vi "run_database.vi"() -> ()   [LabVIEW 2011]
uses:
  <vilib>/addons/database/Connection.llb/DB Tools Open Connec (String).vi
  Dependencies/global.vi
  <vilib>/addons/database/NI_Database_API.lvlib
panel:
  out "Connection Error 4":errorcluster
  out "# Received Data from weather_station.vi":u64
  out "LabVIEW Started at":string
  out "Database Backup Path (remote PC)":path
  out "Backup Error Msg (remote PC)":string
  out "In Progress":bool
  out "Connection Error 3":errorcluster
  out "# Received Data from counter.vi":u64
  out "Dequeue Rate (per second)":dbl
  out "# Elements in Real-time Queue":u64
  out "# Received Data from plc.vi":u64
  out "Connection Error 2":errorcluster
  out "# of Dequeues (total)":u64
  in  "Pause Database Writing (s)":dbl=5.0
  in  "Backup Interval (hour)":dbl=24.0
  out "Backup Error Msg (local PC)":string
  out "Database Backup Path (local PC)":path
  out "Dequeue Paused":bool
  out "# of Backups":u64
  out "Next Backup Dues in (s):":u64 caption="Elapsed Time (s)"
  out "Database Path":path
  out "# Elements in Database Queue":u64
  out "Dequeue Error":errorcluster
  out "Database Access Error":errorcluster
  out "# Received Data from mote.vi":u64
  out "Connection Error":errorcluster
  # "Receive data from motes and Enqueue"
  # "Dequeue and write to database"
  # "Backup database"
  # "Receive data from plcs and Enqueue"
  # "Receive data from people counter and Enqueue"
  # "Receive data from weather station"
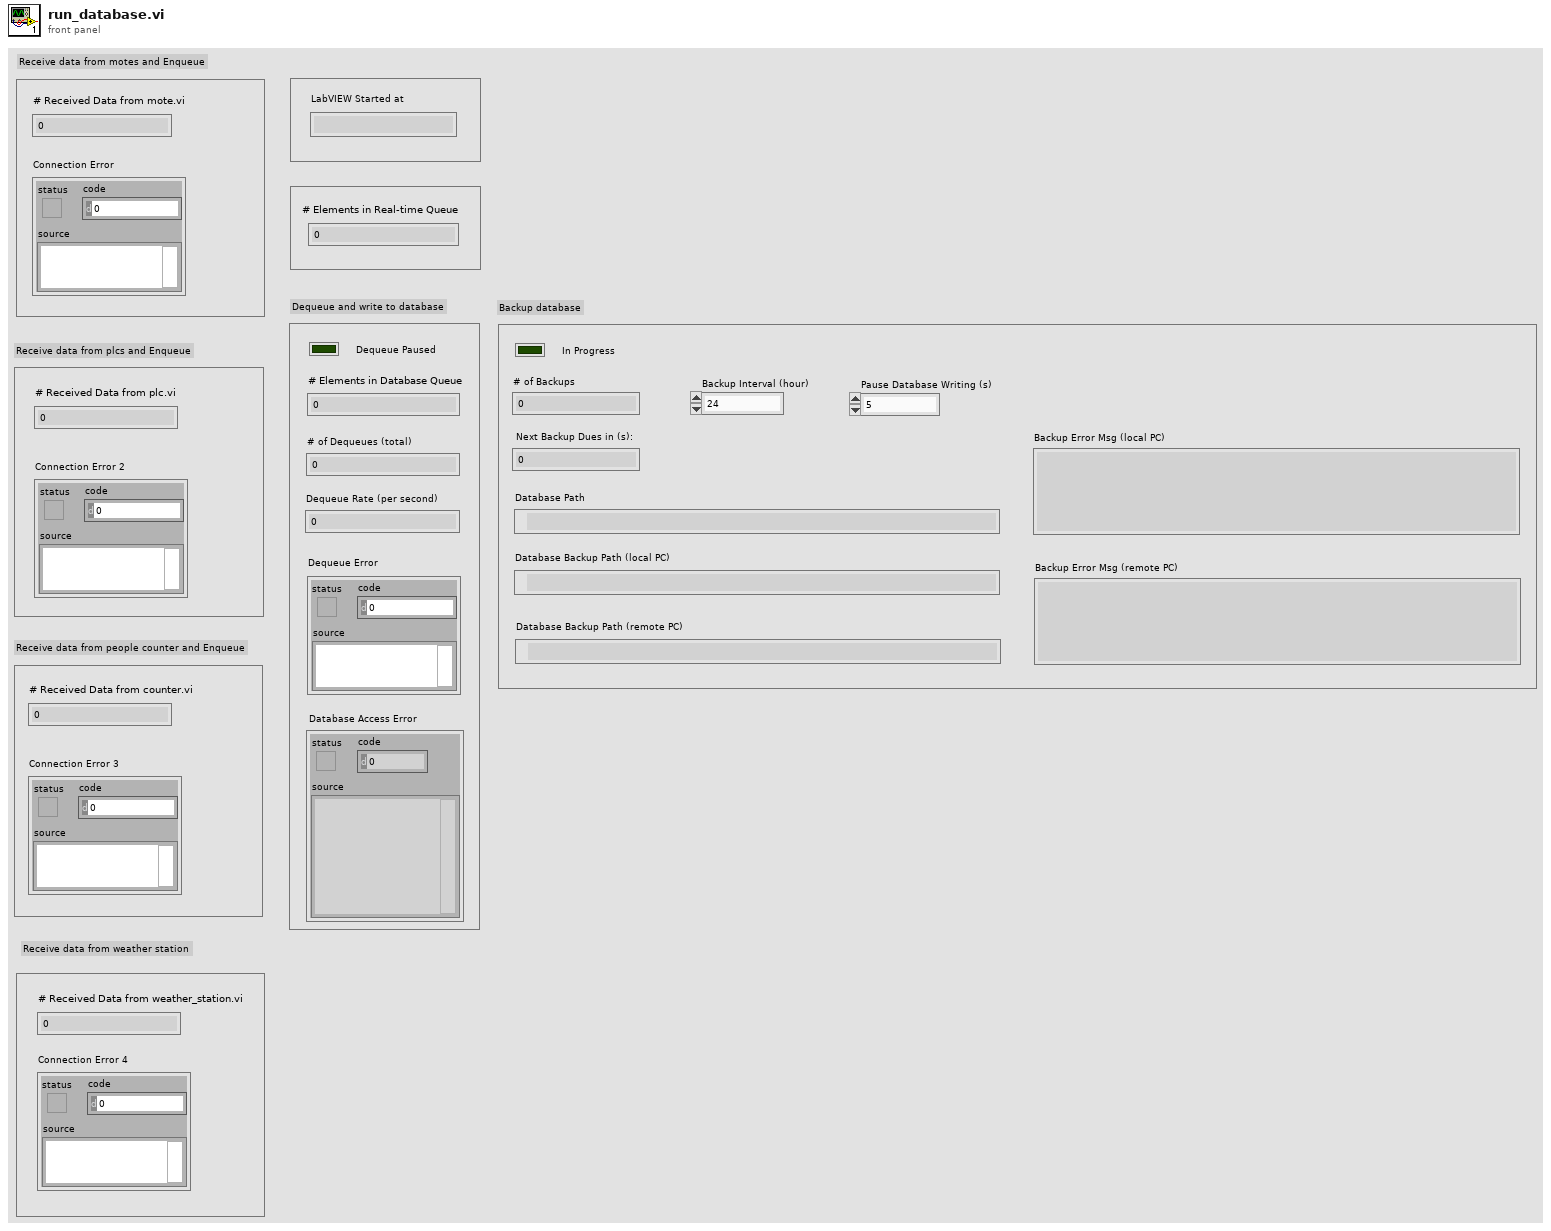
[diagram p1: front panel]
types:
  T1 = enum16{"Read", "Write", "ReadWrite", "BufferedRead", "BufferedReadWrite"}
  T2 = cluster{string, string, string, string, string, string, string, string}
  T3 = cluster{string, "output string":string, "output string":string, "output string":string, "output string":string, "output string":string, "output string":string, "output string":string}
  T4 = typedef "NI_Database_API.lvlib/Conn ObjectReference.ctl" = refnum<k1>
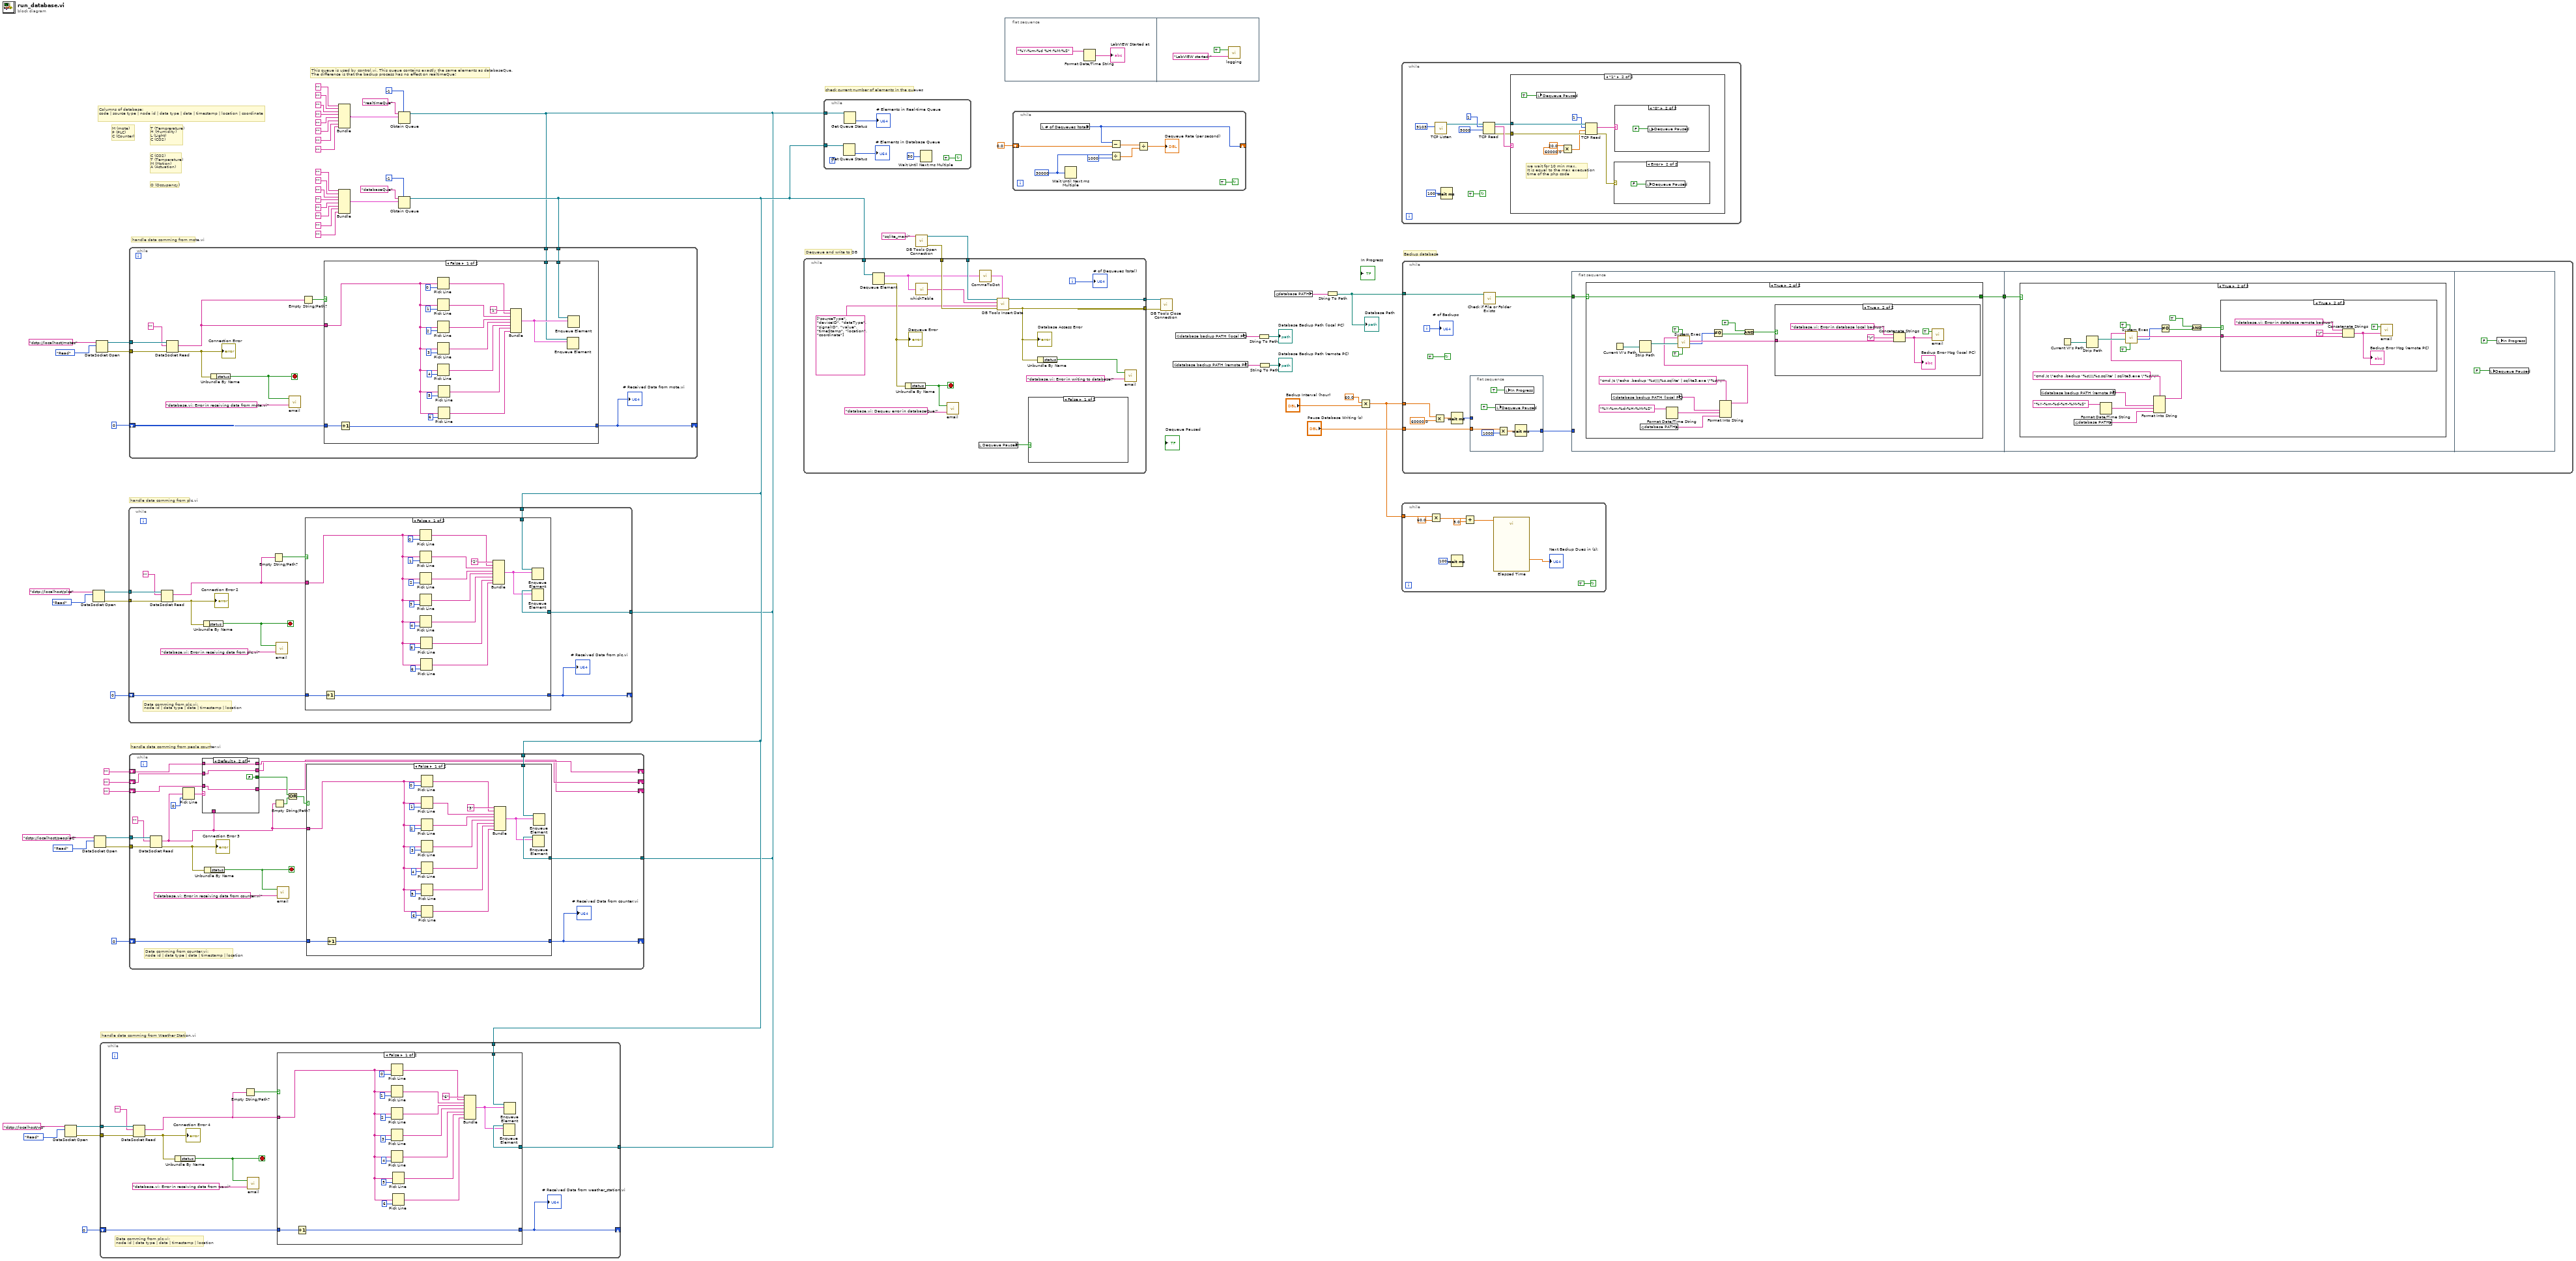
[diagram p0: block diagram]
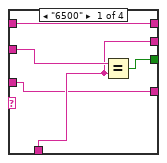
[diagram p6: hidden frame]
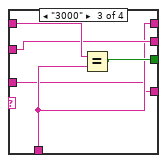
[diagram p7: hidden frame]
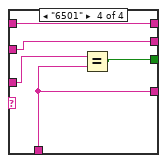
[diagram p8: hidden frame]
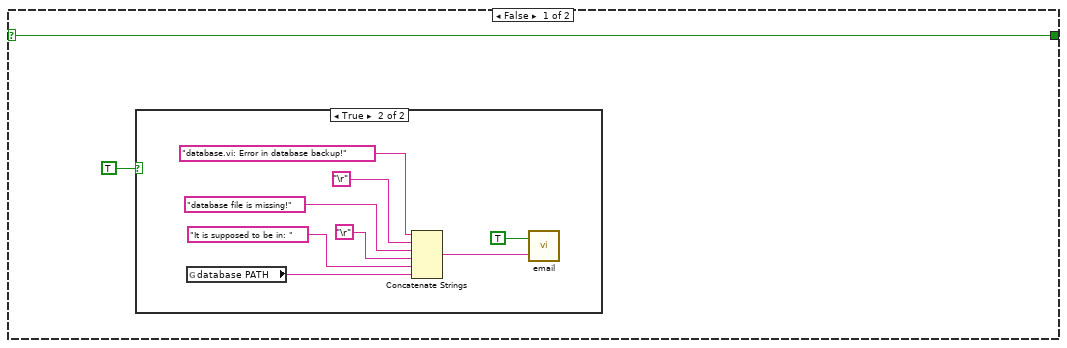
[diagram p11: hidden frame]
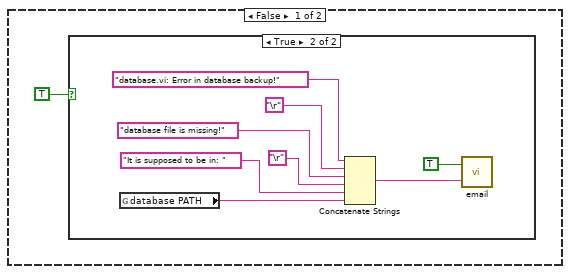
[diagram p14: hidden frame]
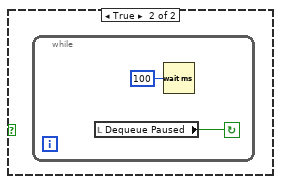
[diagram p17: hidden frame]
diagram:
  # "handle data comming from Weather Station.vi"
  # "handle data comming from peole counter.vi"
  # "O (Occupancy)"
  # "C (CO2)\nT (Temperature)\nM (Motion)\nA (Actuation)"
  # "This queue is used by control.vi. This queue contains exactly the same elements as databaseQue.\nThe difference is that the backup process has no effect on realtimeQue!"
  # "handle data comming from plc.vi"
  # "handle data comming from mote.vi"
  # "Backup database"
  # "Dequeue and write to DB"
  # "check current number of elements in the queues"
  # "M (mote)\nP (PLC)\nC (Counter)"
  # "T (Temprerature)\nH (Humidity)\nL (Light)\nC (CO2)"
  # "Columns of database:\ncode | source type | node id | data type | data | timestamp | location | coordinate"
  n1 = DataSocket Open(10:T1."Read" ("mode"), 11:"dstp://localhost/ws" ("URL 3")) -> (0:w5:errorcluster, 3:w4:refnum<k13>)  [unwired: 2 in]
  n2 = DataSocket Open(10:T1."Read" ("mode"), 11:"dstp://localhost/plcs" ("URL 3")) -> (0:w46:errorcluster, 3:w45:refnum<k13>)  [unwired: 2 in]
  n3 = DataSocket Open(10:T1."Read" ("mode"), 11:"dstp://localhost/peopleC" ("URL 3")) -> (0:w37:errorcluster, 3:w38:refnum<k13>)  [unwired: 2 in]
  n4 = DataSocket Open(10:T1."Read" ("mode"), 11:"dstp://localhost/motes" ("URL 3")) -> (0:w50:errorcluster, 3:w49:refnum<k13>)  [unwired: 2 in]
  n5 = Bundle("", "", "", "", "", "", "", "") -> (w14:T2)  [unwired: 1 in]
  n6 = Bundle("", "", "", "", "", "", "", "") -> (w13:T2)  [unwired: 1 in]
  n7 = Obtain Queue(max queue size (-1, unlimited)=-1, name (unnamed)="realtimeQue", element data type=w14) -> (queue out=w1:refnum<queue>)  [unwired: 2 in, 2 out]
  n8 = Obtain Queue(max queue size (-1, unlimited)=-1, name (unnamed)="databaseQue", element data type=w13) -> (queue out=w2:refnum<queue>)  [unwired: 2 in, 2 out]
  n9 = while {
    tunnel: w5 -> [w75]
    tunnel: w4 -> [w74]
    tunnel: w2 -> [w72]
    tunnel: w1 -> [w70]
    shift-right: [w65] -> _
    shift-left: u64 0 -> [w66]
    stop <- w67 stop-if-true
    # "Data comming from plc.vi:\nnode id | data type | data | timestamp | location"
    n10 = DataSocket Read(8:w75, 10:"", 11:w74) -> (0:w73:errorcluster, 2:w68:string)  [unwired: 2 in, 5 out]
    "Connection Error 4" <- w73
    n11 = Unbundle By Name(w73) -> ("status"=w67:bool)
    n12 = Empty String/Path?(string/path=w68) -> (empty?=w69:bool)
    n13 = call "email.vi"("Body"="database.vi: Error in receiving data from ws.vi", "Enable"=w67) -> ()  [unwired: 1 in]
    n14 = case shown="False" w69 {
      tunnel: w72 -> [w96 _]
      tunnel: w68 -> [w80 _]
      tunnel: w70 -> [w90 _]
      tunnel: w66 -> [w88 w97]
      tunnel: [w87 w97] -> w65
      frame False {
        n15 = Increment(x=w88) -> (x+1=w87:u64)
        n16 = Pick Line(multi-line string=w80, line index=0) -> (output string=w76:string)  [unwired: 1 in]
        n17 = Pick Line(multi-line string=w80, line index=1) -> (output string=w86:string)  [unwired: 1 in]
        n18 = Pick Line(multi-line string=w80, line index=2) -> (output string=w85:string)  [unwired: 1 in]
        n19 = Pick Line(multi-line string=w80, line index=3) -> (output string=w84:string)  [unwired: 1 in]
        n20 = Pick Line(multi-line string=w80, line index=4) -> (output string=w83:string)  [unwired: 1 in]
        n21 = Pick Line(multi-line string=w80, line index=5) -> (output string=w79:string)  [unwired: 1 in]
        n22 = Pick Line(multi-line string=w80, line index=6) -> (output string=w78:string)  [unwired: 1 in]
        n23 = Bundle("6", "output string"=w76, "output string"=w86, "output string"=w85, "output string"=w84, "output string"=w83, "output string"=w79, "output string"=w78) -> (w89:T3)  [unwired: 1 in]
        n24 = Enqueue Element(queue=w90, element=w89) -> ()  [unwired: 2 in, 3 out]
        n25 = Enqueue Element(queue=w96, element=w89) -> ()  [unwired: 2 in, 3 out]
      }
      frame True {
      }
    }
    "# Received Data from weather_station.vi" <- w65
  }
  n26 = while {
    tunnel: w46 -> [w109]
    tunnel: w45 -> [w108]
    tunnel: w2 -> [w106]
    tunnel: w1 -> [w104]
    shift-right: [w99] -> _
    shift-left: u64 0 -> [w100]
    stop <- w101 stop-if-true
    # "Data comming from plc.vi:\nnode id | data type | data | timestamp | location"
    n27 = DataSocket Read(8:w109, 10:"", 11:w108) -> (0:w107:errorcluster, 2:w102:string)  [unwired: 2 in, 5 out]
    "Connection Error 2" <- w107
    n28 = Unbundle By Name(w107) -> ("status"=w101:bool)
    n29 = Empty String/Path?(string/path=w102) -> (empty?=w103:bool)
    n30 = call "email.vi"("Body"="database.vi: Error in receiving data from plc.vi", "Enable"=w101) -> ()  [unwired: 1 in]
    n31 = case shown="False" w103 {
      tunnel: w106 -> [w130 _]
      tunnel: w102 -> [w114 _]
      tunnel: w104 -> [w124 _]
      tunnel: w100 -> [w122 w131]
      tunnel: [w121 w131] -> w99
      frame False {
        n32 = Increment(x=w122) -> (x+1=w121:u64)
        n33 = Pick Line(multi-line string=w114, line index=0) -> (output string=w110:string)  [unwired: 1 in]
        n34 = Pick Line(multi-line string=w114, line index=1) -> (output string=w120:string)  [unwired: 1 in]
        n35 = Pick Line(multi-line string=w114, line index=2) -> (output string=w119:string)  [unwired: 1 in]
        n36 = Pick Line(multi-line string=w114, line index=3) -> (output string=w118:string)  [unwired: 1 in]
        n37 = Pick Line(multi-line string=w114, line index=4) -> (output string=w117:string)  [unwired: 1 in]
        n38 = Pick Line(multi-line string=w114, line index=5) -> (output string=w113:string)  [unwired: 1 in]
        n39 = Pick Line(multi-line string=w114, line index=6) -> (output string=w112:string)  [unwired: 1 in]
        n40 = Bundle("2", "output string"=w110, "output string"=w120, "output string"=w119, "output string"=w118, "output string"=w117, "output string"=w113, "output string"=w112) -> (w123:T3)  [unwired: 1 in]
        n41 = Enqueue Element(queue=w124, element=w123) -> ()  [unwired: 2 in, 3 out]
        n42 = Enqueue Element(queue=w130, element=w123) -> ()  [unwired: 2 in, 3 out]
      }
      frame True {
      }
    }
    "# Received Data from plc.vi" <- w99
  }
  n43 = while {
    tunnel: w50 -> [w143]
    tunnel: w49 -> [w142]
    tunnel: w2 -> [w140]
    tunnel: w1 -> [w139]
    shift-right: [w136] -> _
    shift-left: u64 0 -> [w137]
    stop <- w138 stop-if-true
    n44 = DataSocket Read(8:w143, 10:"", 11:w142) -> (0:w141:errorcluster, 2:w132:string)  [unwired: 2 in, 5 out]
    "Connection Error" <- w141
    n45 = Unbundle By Name(w141) -> ("status"=w138:bool)
    n46 = call "email.vi"("Body"="database.vi: Error in receiving data from mote.vi", "Enable"=w138) -> ()  [unwired: 1 in]
    n47 = Empty String/Path?(string/path=w132) -> (empty?=w134:bool)
    n48 = case shown="False" w134 {
      tunnel: w140 -> [w148 _]
      tunnel: w132 -> [w146 _]
      tunnel: w139 -> [w147 _]
      tunnel: [w164 w165] -> w136
      tunnel: w137 -> [w163 w165]
      frame False {
        n49 = Increment(x=w163) -> (x+1=w164:u64)
        n50 = Pick Line(multi-line string=w146, line index=0) -> (output string=w144:string)  [unwired: 1 in]
        n51 = Pick Line(multi-line string=w146, line index=1) -> (output string=w156:string)  [unwired: 1 in]
        n52 = Pick Line(multi-line string=w146, line index=2) -> (output string=w155:string)  [unwired: 1 in]
        n53 = Pick Line(multi-line string=w146, line index=3) -> (output string=w154:string)  [unwired: 1 in]
        n54 = Pick Line(multi-line string=w146, line index=4) -> (output string=w153:string)  [unwired: 1 in]
        n55 = Pick Line(multi-line string=w146, line index=5) -> (output string=w150:string)  [unwired: 1 in]
        n56 = Pick Line(multi-line string=w146, line index=6) -> (output string=w149:string)  [unwired: 1 in]
        n57 = Bundle("1", "output string"=w144, "output string"=w156, "output string"=w155, "output string"=w154, "output string"=w153, "output string"=w150, "output string"=w149) -> (w157:T3)  [unwired: 1 in]
        n58 = Enqueue Element(queue=w147, element=w157) -> ()  [unwired: 2 in, 3 out]
        n59 = Enqueue Element(queue=w148, element=w157) -> ()  [unwired: 2 in, 3 out]
      }
      frame True {
      }
    }
    "# Received Data from mote.vi" <- w136
  }
  n60 = while {
    tunnel: w37 -> [w187]
    tunnel: w38 -> [w186]
    tunnel: w2 -> [w184]
    tunnel: w1 -> [w182]
    shift-right: [w179] -> _
    shift-left: u64 0 -> [w180]
    shift-right: [w169] -> _
    shift-left: "" -> [w173]
    shift-right: [w168] -> _
    shift-left: "" -> [w170]
    shift-right: [w166] -> _
    shift-left: "" -> [w167]
    stop <- w181 stop-if-true
    # "Data comming from counter.vi:\nnode id | data type | data | timestamp | location"
    n61 = DataSocket Read(8:w187, 10:"", 11:w186) -> (0:w185:errorcluster, 2:w172:string)  [unwired: 2 in, 5 out]
    "Connection Error 3" <- w185
    n62 = Pick Line(multi-line string=w172, line index=0) -> (output string=w174:string)  [unwired: 1 in]
    n63 = case shown="Default" w174 {
      tunnel: w173 -> [w191 w196 w200 w204]
      tunnel: w172 -> [w189 _ w198 w202]
      tunnel: [w192 FALSE w201 w206] -> w171
      tunnel: w170 -> [w190 w195 w199 w205]
      tunnel: [w191 w196 w198 w204] -> w169
      tunnel: [w189 w195 w199 w205] -> w168
      tunnel: w167 -> [w188 w193 w197 w203]
      tunnel: [w188 w193 w197 w202] -> w166
      frame "6500" {
        n64 = Equal?(x=w190, y=w189) -> (x = y?=w192:bool)
      }
      frame Default {
      }
      frame "3000" {
        n65 = Equal?(x=w200, y=w198) -> (x = y?=w201:bool)
      }
      frame "6501" {
        n66 = Equal?(x=w203, y=w202) -> (x = y?=w206:bool)
      }
    }
    n67 = Unbundle By Name(w185) -> ("status"=w181:bool)
    n68 = Empty String/Path?(string/path=w172) -> (empty?=w177:bool)
    n69 = call "email.vi"("Body"="database.vi: Error in receiving data from counter.vi", "Enable"=w181) -> ()  [unwired: 1 in]
    n70 = Or(x=w171, y=w177) -> (x .or. y?=w176:bool)
    n71 = case shown="False" w176 {
      tunnel: w184 -> [w227 _]
      tunnel: w172 -> [w211 _]
      tunnel: w182 -> [w221 _]
      tunnel: w180 -> [w219 w228]
      tunnel: [w218 w228] -> w179
      frame False {
        n72 = Increment(x=w219) -> (x+1=w218:u64)
        n73 = Pick Line(multi-line string=w211, line index=0) -> (output string=w207:string)  [unwired: 1 in]
        n74 = Pick Line(multi-line string=w211, line index=1) -> (output string=w217:string)  [unwired: 1 in]
        n75 = Pick Line(multi-line string=w211, line index=2) -> (output string=w216:string)  [unwired: 1 in]
        n76 = Pick Line(multi-line string=w211, line index=3) -> (output string=w215:string)  [unwired: 1 in]
        n77 = Pick Line(multi-line string=w211, line index=4) -> (output string=w214:string)  [unwired: 1 in]
        n78 = Pick Line(multi-line string=w211, line index=5) -> (output string=w210:string)  [unwired: 1 in]
        n79 = Pick Line(multi-line string=w211, line index=6) -> (output string=w209:string)  [unwired: 1 in]
        n80 = Bundle("3", "output string"=w207, "output string"=w217, "output string"=w216, "output string"=w215, "output string"=w214, "output string"=w210, "output string"=w209) -> (w220:T3)  [unwired: 1 in]
        n81 = Enqueue Element(queue=w221, element=w220) -> ()  [unwired: 2 in, 3 out]
        n82 = Enqueue Element(queue=w227, element=w220) -> ()  [unwired: 2 in, 3 out]
      }
      frame True {
      }
    }
    "# Received Data from counter.vi" <- w179
  }
  n83 = while {
    tunnel: w2 -> [w234]
    tunnel: w1 -> [w230]
    stop <- TRUE continue-if-true
    n84 = Get Queue Status(queue=w234) -> (# elements in queue=→"# Elements in Database Queue":i32)  [unwired: 2 in, 7 out]
    n85 = Get Queue Status(queue=w230) -> (# elements in queue=→"# Elements in Real-time Queue":i32)  [unwired: 2 in, 7 out]
    n86 = Wait Until Next ms Multiple(millisecond multiple=u32 50) -> ()  [unwired: 1 out]
  }
  n87 = call-poly <vilib>:"DB Tools Open Connection.vi"("connection information"="sqlite_mani") -> ("error out"=w56:errorcluster, "connection reference"=w59:T4)  [unwired: 7 in]
  n88 = while {
    tunnel: w59 -> [w249]
    tunnel: [w250] -> w58
    tunnel: [w240] -> w57
    tunnel: w56 -> [w248]
    tunnel: w2 -> [w247]
    i -> [w243]
    stop <- w241 stop-if-true
    n89 = Dequeue Element(queue=w247) -> (element=w236:T2, error out=w246:errorcluster)  [unwired: 2 in, 2 out]
    "Dequeue Error" <- w246
    n90 = Unbundle By Name(w246) -> ("status"=w241:bool)
    n91 = call "whichTable.vi"("output cluster"=w236) -> ("String"=w242:string)
    n92 = call "email.vi"("Body"="database.vi: Dequeu error in databaseQue!", "Enable"=w241) -> ()  [unwired: 1 in]
    n93 = local read "Dequeue Paused"() -> (w244:bool)
    n94 = call "CommaToDot.vi"("Input"=w236) -> ("Output"=w235:T2)
    n95 = call <vilib>:"DB Tools Insert Data.vi"("data"=w235, "error in (no error)"=w248, "columns"=string[] ["sourceType", "deviceID", "dataType", "signalID", "value", "timeStamp", "location", "coordinate"], "table"=w242, "connection reference"=w249) -> ("error out"=w240:errorcluster, "connection reference out"=w250:T4)  [unwired: 5 in]
    "Database Access Error" <- w240
    n96 = case shown="False" w244 {
      frame False {
      }
      frame True {
        n97 = while {
          stop <- w251 continue-if-true
          n98 = local read "Dequeue Paused"() -> (w251:bool)
          n99 = Wait (ms)(milliseconds to wait=u32 100) -> ()  [unwired: 1 out]
        }
      }
    }
    n100 = Unbundle By Name(w240) -> ("status"=w239:bool)
    n101 = call "email.vi"("Body"="database.vi: Error in writing to database!", "Enable"=w239) -> ()  [unwired: 1 in]
    "# of Dequeues (total)" <- w243
  }
  n102 = flat-sequence {
    frame #0 {
      n103 = Format Date/Time String(time format string (%c)="%Y-%m-%d %H:%M:%S") -> (date/time string=→"LabVIEW Started at":string)  [unwired: 2 in]
    }
    frame #1 {
      n104 = call "logging.vi"("data"="LabVIEW started.", "Boolean"=TRUE) -> ()  [unwired: 1 in]
    }
  }
  n105 = while {
    shift-right: [w262] -> _
    shift-left: 0.0 -> [w263]
    stop <- TRUE continue-if-true
    w259 = u32 30000 ("millisecond multiple")
    n106 = local read "# of Dequeues (total)"() -> (w262:u64)
    n107 = Wait Until Next ms Multiple(millisecond multiple=w259) -> ()  [unwired: 1 out]
    n108 = Subtract(x=w262, y=w263) -> (x-y=w261:dbl)
    n109 = Divide(x=w259, y=u32 1000) -> (x/y=w257:dbl)
    n110 = Divide(x=w261, y=w257) -> (x/y=→"Dequeue Rate (per second)":dbl)
  }
  n111 = call <vilib>:"DB Tools Close Connection.vi"("error in (no error)"=w57, "connection reference"=w58) -> ()  [unwired: 5 in, 1 out]
  n112 = global read "global.vi" "database backup PATH (remote PC)"() -> (w11:string)
  n113 = global read "global.vi" "database backup PATH (local PC)"() -> (w53:string)
  n114 = String To Path(string=w53) -> (path=→"Database Backup Path (local PC)":path)
  n115 = String To Path(string=w11) -> (path=→"Database Backup Path (remote PC)":path)
  n116 = global read "global.vi" "database PATH"() -> (w55:string)
  n117 = String To Path(string=w55) -> (path=w54:path)
  "Database Path" <- w54
  n118 = Multiply(x=60.0, y="Backup Interval (hour)") -> (x*y=w31:dbl)
  n119 = while {
    stop <- TRUE continue-if-true
    n120 = call <vilib>:"TCP Listen.vi"("port"=u16 9103) -> ("connection ID"=w268:refnum<k5>)  [unwired: 6 in, 4 out]
    n121 = Wait (ms)(milliseconds to wait=u32 100) -> ()  [unwired: 1 out]
    n122 = TCP Read(connection ID=w268, bytes to read=1, 9:5000 ("timeout ms (25000)")) -> (connection ID out=w266:refnum<k5>, data out=w267:string, error out=w265:errorcluster)  [unwired: 2 in]
    n123 = case shown="\"1\"" w267 {
      tunnel: w266 -> [_ w282]
      tunnel: w265 -> [_ w281]
      frame "0", Default {
      }
      frame "1" {
        # "we wait for 10 min max.\nIt is equal to the max execuation\ntime of the php code"
        n124 = local write "Dequeue Paused"(TRUE ("Backup in Progress")) -> ()
        n125 = Multiply(x=20.0, y=60000.0) -> (x*y=w274:dbl)
        n126 = TCP Read(connection ID=w282, bytes to read=1, error in (no error)=w281, 9:w274) -> (data out=w278:string, error out=w277:errorcluster)  [unwired: 1 in, 1 out]
        n127 = case shown="Error" w277 {
          frame No Error {
          }
          frame Error {
            n128 = local write "Dequeue Paused"(FALSE ("Backup in Progress")) -> ()
          }
        }
        n129 = case shown="\"0\"" w278 {
          frame "1", Default {
          }
          frame "0" {
            n130 = local write "Dequeue Paused"(FALSE ("Backup in Progress")) -> ()
          }
        }
      }
    }
  }
  n131 = while {
    tunnel: w31 -> [w290]
    stop <- TRUE continue-if-true
    n132 = Multiply(x=w290, y=60.0) -> (x*y=w287:dbl)
    n133 = Wait (ms)(milliseconds to wait=u32 100) -> ()  [unwired: 1 out]
    n134 = Add(x=w287, y=5.0) -> (x+y=w288:dbl)
    n135 = call "Elapsed Time"("Time Target (s)"=w288) -> ("Elapsed Time (s)"=→"Next Backup Dues in (s):":dbl)  [unwired: 11 in, 7 out]
  }
  n136 = while {
    tunnel: w54 -> [w302]
    tunnel: w31 -> [w296]
    tunnel: "Pause Database Writing (s)" -> [w295]
    i -> [w294]
    stop <- TRUE continue-if-true
    n137 = Multiply(x=w296, y=60000.0) -> (x*y=w297:dbl)
    n138 = Wait (ms)(milliseconds to wait=w297) -> (millisecond timer value=w301:u32)
    n139 = flat-sequence {
      tunnel: w301 -> [_]
      tunnel: [w309] -> w300
      tunnel: w295 -> [w307]
      frame #0 {
        n140 = local write "Dequeue Paused"(TRUE ("Pause Write to DB")) -> ()
        n141 = Multiply(x=w307, y=u32 1000) -> (x*y=w308:dbl)
        n142 = local write "In Progress"(TRUE ("In Progress")) -> ()
        n143 = Wait (ms)(milliseconds to wait=w308) -> (millisecond timer value=w309:u32)
      }
    }
    n144 = call <vilib>:"Check if File or Folder Exists.vi"("path"=w302) -> ("file or folder exists?"=w298:bool)  [unwired: 8 in, 2 out]
    n145 = flat-sequence {
      tunnel: w300 -> [_]
      tunnel: w298 -> [w311]
      tunnel: [w310] -> w293
      tunnel: w293 -> [w343]
      frame #0 {
        n146 = case shown="True" w311 {
          selector: w311 -> [w312 w322]
          tunnel: [w312 w322] -> w310
          frame False {
            n147 = case shown="True" TRUE {
              frame False {
              }
              frame True {
                n148 = global read "global.vi" "database PATH"() -> (w316:string)
                n149 = Concatenate Strings("database.vi: Error in database backup!", "\r", "database file is missing!", "\r", "It is supposed to be in: ", w316) -> (w314:string)
                n150 = call "email.vi"("Body"=w314, "Enable"=TRUE) -> ()  [unwired: 1 in]
              }
            }
          }
          frame True {
            n151 = global read "global.vi" "database backup PATH (local PC)"() -> (w326:string)
            n152 = Current VI's Path() -> (path=w333:path)
            n153 = Strip Path(path=w333) -> (stripped path=w332:path)  [unwired: 1 out]
            n154 = global read "global.vi" "database PATH"() -> (w328:string)
            n155 = Format Date/Time String(time format string (%c)="%Y-%m-%d-%H-%M-%S") -> (date/time string=w327:string)  [unwired: 2 in]
            n156 = Format Into String(format string="cmd /c \"echo .backup '%s\\\\%s.sqlite' | sqlite3.exe \"%s\"\"", w326, w327, w328) -> (resulting string=w323:string)  [unwired: 2 in, 1 out]
            n157 = call <vilib>:"System Exec.vi"("run minimized? (F)"=TRUE, "wait until completion? (T)"=TRUE, "working directory"=w332, "command line"=w323) -> ("return code"=w330:i32, "standard error"=w331:string)  [unwired: 4 in, 2 out]
            n158 = Not Equal To 0?(x=w330) -> (x != 0?=w329:bool)
            n159 = And(x=TRUE, y=w329) -> (x .and. y?=w337:bool)
            n160 = case shown="True" w337 {
              tunnel: w331 -> [_ w340]
              frame False {
              }
              frame True {
                n161 = Concatenate Strings("database.vi: Error in database local backup!", "\r", w340) -> (w338:string)
                "Backup Error Msg (local PC)" <- w338
                n162 = call "email.vi"("Body"=w338, "Enable"=TRUE) -> ()  [unwired: 1 in]
              }
            }
          }
        }
      }
      frame #1 {
        n163 = case shown="True" w343 {
          frame False {
            n164 = case shown="True" TRUE {
              frame False {
              }
              frame True {
                n165 = global read "global.vi" "database PATH"() -> (w347:string)
                n166 = Concatenate Strings("database.vi: Error in database backup!", "\r", "database file is missing!", "\r", "It is supposed to be in: ", w347) -> (w345:string)
                n167 = call "email.vi"("Body"=w345, "Enable"=TRUE) -> ()  [unwired: 1 in]
              }
            }
          }
          frame True {
            n168 = global read "global.vi" "database backup PATH (remote PC)"() -> (w356:string)
            n169 = Current VI's Path() -> (path=w363:path)
            n170 = global read "global.vi" "database PATH"() -> (w358:string)
            n171 = Strip Path(path=w363) -> (stripped path=w362:path)  [unwired: 1 out]
            n172 = Format Date/Time String(time format string (%c)="%Y-%m-%d-%H-%M-%S") -> (date/time string=w357:string)  [unwired: 2 in]
            n173 = Format Into String(format string="cmd /c \"echo .backup '%s\\\\%s.sqlite' | sqlite3.exe \"%s\"\"", w356, w357, w358) -> (resulting string=w353:string)  [unwired: 2 in, 1 out]
            n174 = call <vilib>:"System Exec.vi"("run minimized? (F)"=TRUE, "wait until completion? (T)"=TRUE, "working directory"=w362, "command line"=w353) -> ("return code"=w360:i32, "standard error"=w361:string)  [unwired: 4 in, 2 out]
            n175 = Not Equal To 0?(x=w360) -> (x != 0?=w359:bool)
            n176 = And(x=TRUE, y=w359) -> (x .and. y?=w367:bool)
            n177 = case shown="True" w367 {
              tunnel: w361 -> [_ w370]
              frame False {
              }
              frame True {
                n178 = Concatenate Strings("database.vi: Error in database remote backup!", "\r", w370) -> (w368:string)
                "Backup Error Msg (remote PC)" <- w368
                n179 = call "email.vi"("Body"=w368, "Enable"=TRUE) -> ()  [unwired: 1 in]
              }
            }
          }
        }
      }
      frame #2 {
        n180 = local write "Dequeue Paused"(FALSE ("Pause Write to DB")) -> ()
        n181 = local write "In Progress"(FALSE ("In Progress")) -> ()
      }
    }
    "# of Backups" <- w294
  }
